vi "Prober_MoveToLoad.vi"(8 "error in (no error)":errorcluster, 11 "SemiProbe in":refnum<class "SemiProbe.lvclass">) -> (0 "error out":errorcluster, 3 "SemiProbe out":refnum<class "SemiProbe.lvclass">)   [LabVIEW 2013, in "SemiProbe.lvclass"]
uses:
  SemiProbe.lvclass
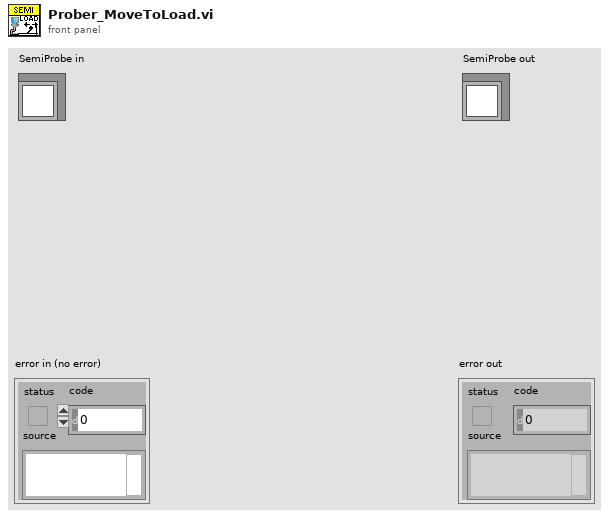
[diagram p1: front panel]
types:
  T1 = enum16{"Move To Load", "Move To Double Separation", "Move To Separation Distance", "Move To Contact", "Execute Contact Search", "Execute Arduino Contact Search"}
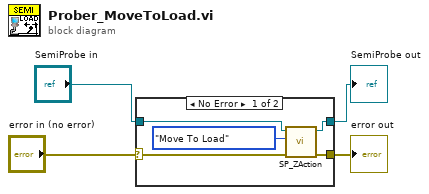
[diagram p0: block diagram]
diagram:
  n1 = case shown="No Error" "error in (no error)" {
    selector: "error in (no error)" -> [w7 w10]
    tunnel: "SemiProbe in" -> [w8 w11]
    tunnel: [w5 w11] -> w3
    tunnel: [w6 w10] -> w1
    frame No Error {
      n2 = call-dynamic "SP_ZAction.vi"("error in (no error)"=w7, "Z Action"=T1."Move To Load", "SemiProbe in"=w8) -> ("error out"=w6:errorcluster, "SemiProbe out"=w5:refnum<class "SemiProbe.lvclass">)  [unwired: 5 in, 2 out]
    }
    frame Error {
    }
  }
  "error out" <- w1
  "SemiProbe out" <- w3
